vi "Status.vi"() -> ()   [LabVIEW 2013]
uses:
  Arm Globals.vi
  ROS/Code/Console/Servers/ServerSubs/(nist) Arm Globals.vi
panel:
  out "L: End":bool caption="Abort"
  out "L: Pause":bool caption="Pause"
  out "L: Status":string="Initial" caption="Prim Status"
  in  "Use Through Point":bool=TRUE
  in  "Zero V":bool
  out "R: End":bool caption="Abort"
  out "R: Pause":bool caption="Pause"
  in  "stop":bool
  out "R:Status":string="Home" caption="Prim Status"
  # "Right"
  # "Left"
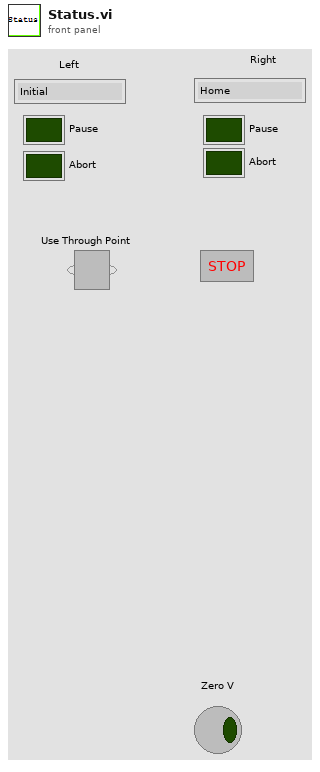
[diagram p1: front panel]
types:
  T1 = cluster{"Label":string, "Arm Angles (degrees)":dbl[]}
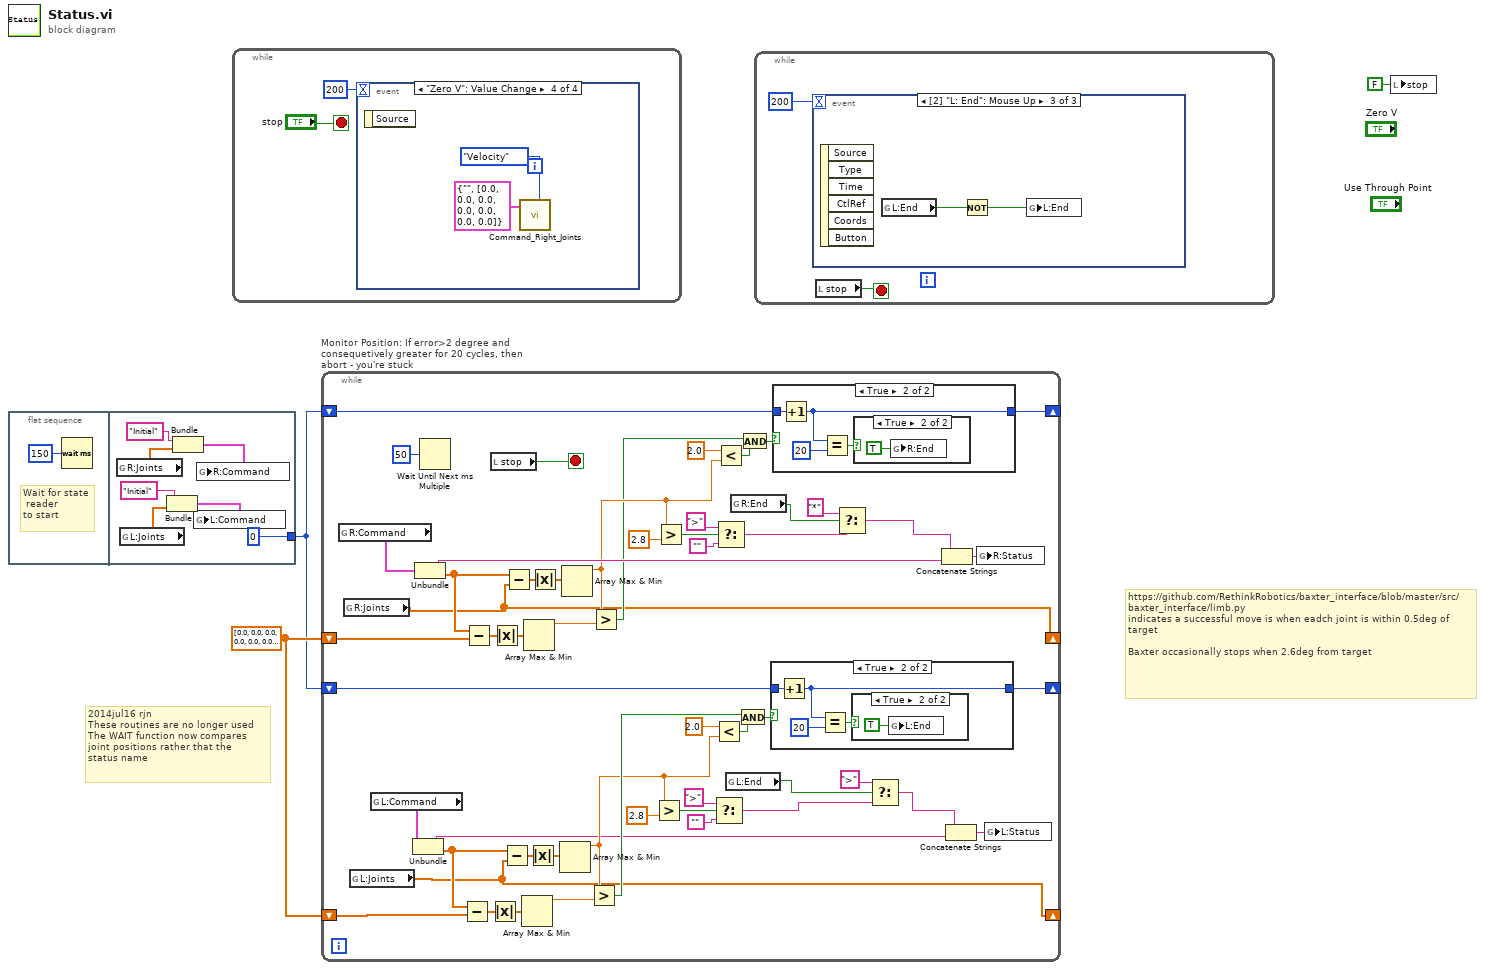
[diagram p0: block diagram]
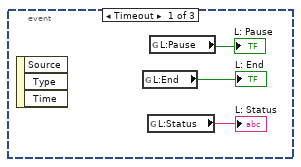
[diagram p2: hidden frame]
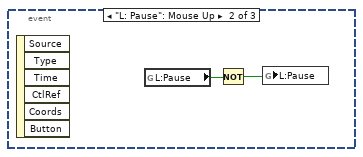
[diagram p3: hidden frame]
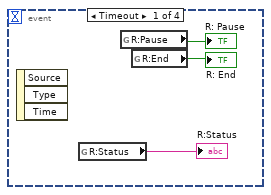
[diagram p4: hidden frame]
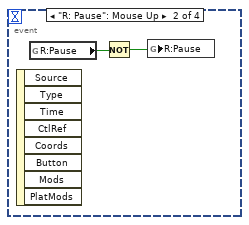
[diagram p5: hidden frame]
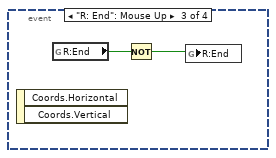
[diagram p6: hidden frame]
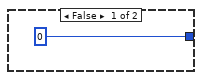
[diagram p7: hidden frame]
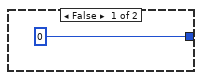
[diagram p9: hidden frame]
diagram:
  w2 = dbl[] [0.0, 0.0, 0.0, 0.0, 0.0, 0.0, 0.0] ("Positions")
  # "2014jul16 rjn\nThese routines are no longer used\nThe WAIT function now compares\njoint positions rather that the \nstatus name"
  # "https://github.com/RethinkRobotics/baxter_interface/blob/master/src/baxter_interface/limb.py\nindicates a successful move is when eadch joint is within 0.5deg of target\n\nBaxter occasionally stops when 2.6deg from target"
  n1 = flat-sequence {
    tunnel: [0] -> w1
    frame #0 {
      # "Wait for state\n reader\nto start"
      n2 = Wait (ms)(milliseconds to wait=u32 150) -> ()  [unwired: 1 out]
    }
    frame #1 {
      n3 = global read "(nist) Arm Globals.vi" "R:Joints"() -> (w6:dbl[])
      n4 = global read "(nist) Arm Globals.vi" "L:Joints"() -> (w5:dbl[])
      n5 = Bundle("Initial", "L:Joints"=w5) -> (w7:cluster{string, "L:Joints":dbl[]})  [unwired: 1 in]
      n6 = Bundle("Initial", "R:Joints"=w6) -> (w8:cluster{string, "R:Joints":dbl[]})  [unwired: 1 in]
      n7 = global write "Arm Globals.vi" "L:Command"(w7) -> ()
      n8 = global write "Arm Globals.vi" "R:Command"(w8) -> ()
    }
  }
  n9 = while {
    stop <- "stop" stop-if-true
    n10 = event shown="[3] \"Zero V\": Value Change" {
      selector: _ -> [_ _ _ _]
      dyn-events: _ -> [_ _ _ _]
      timeout: 200 -> [_ _ _ _]
      event Timeout {
        n11 = event-data() -> ()  [unwired: 1 in, 3 out]
        n12 = global read "Arm Globals.vi" "R:Status"() -> (→"R:Status":string)
        n13 = global read "Arm Globals.vi" "R:Pause"() -> (→"R: Pause":bool)
        n14 = global read "Arm Globals.vi" "R:End"() -> (→"R: End":bool)
      }
      event "R: Pause": Mouse Up {
        n15 = event-data() -> ()  [unwired: 1 in, 8 out]
        n16 = global read "Arm Globals.vi" "R:Pause"() -> (w18:bool)
        n17 = Not(x=w18) -> (.not. x?=w17:bool)
        n18 = global write "Arm Globals.vi" "R:Pause"(w17) -> ()
      }
      event "R: End": Mouse Up {
        n19 = event-data() -> ()  [unwired: 1 in, 2 out]
        n20 = global read "Arm Globals.vi" "R:End"() -> (w20:bool)
        n21 = Not(x=w20) -> (.not. x?=w19:bool)
        n22 = global write "Arm Globals.vi" "R:End"(w19) -> ()
      }
      event "Zero V": Value Change {
        n23 = event-data() -> ()  [unwired: 1 in, 1 out]
        n24 = call "Command_Right_Joints.vi"("Mode"=enum32{"Position", "Velocity", "Effort"}."Velocity", "Goal"=T1 {"Label"="", "Arm Angles (degrees)"=[0.0, 0.0, 0.0, 0.0, 0.0, 0.0, 0.0]}) -> ()  [unwired: 6 in, 2 out]
      }
    }
  }
  n25 = while "Monitor Position: If error>2 degree and consequetively greater for 20 cycles, then abort - you're stuck" {
    shift-right: [w73] -> _
    shift-left: w1 -> [w72]
    shift-right: [w24] -> _
    shift-left: w2 -> [w59]
    shift-right: [w35] -> _
    shift-left: w1 -> [w36]
    shift-right: [w23] -> _
    shift-left: w2 -> [w37]
    stop <- w71 stop-if-true
    n26 = global read "Arm Globals.vi" "R:Command"() -> (w26:cluster{"Label":string, "Angles":dbl[]})
    n27 = global read "(nist) Arm Globals.vi" "R:Joints"() -> (w24:dbl[])
    n28 = global read "(nist) Arm Globals.vi" "L:Joints"() -> (w23:dbl[])
    n29 = global read "Arm Globals.vi" "L:Command"() -> (w25:cluster{"Label":string, "Angles":dbl[]})
    n30 = Unbundle(w25) -> ("Label"=w45:string, "Angles"=w50:dbl[])
    n31 = Unbundle(w26) -> ("Label"=w65:string, "Angles"=w60:dbl[])
    n32 = Wait Until Next ms Multiple(millisecond multiple=u32 50) -> ()  [unwired: 1 out]
    n33 = Subtract(x=w50, y=w37) -> (x-y=w51:dbl[])
    n34 = Subtract(x=w60, y=w59) -> (x-y=w58:dbl[])
    n35 = Absolute Value(x=w51) -> (abs(x)=w49:dbl[])
    n36 = local read "stop"() -> (w71:bool)
    n37 = Absolute Value(x=w58) -> (abs(x)=w61:dbl[])
    n38 = Subtract(x=w50, y=w23) -> (x-y=w38:dbl[])
    n39 = Subtract(x=w60, y=w24) -> (x-y=w76:dbl[])
    n40 = Array Max & Min(array=w49) -> (max value=w52:dbl)  [unwired: 3 out]
    n41 = Array Max & Min(array=w61) -> (max value=w57:dbl)  [unwired: 3 out]
    n42 = Absolute Value(x=w38) -> (abs(x)=w40:dbl[])
    n43 = Absolute Value(x=w76) -> (abs(x)=w70:dbl[])
    n44 = Array Max & Min(array=w40) -> (max value=w53:dbl)  [unwired: 3 out]
    n45 = Array Max & Min(array=w70) -> (max value=w56:dbl)  [unwired: 3 out]
    n46 = Greater?(x=w53, y=w52) -> (0:w54:bool)
    n47 = Greater?(x=w56, y=w57) -> (0:w55:bool)
    n48 = Greater?(x=w53, y=2.8) -> (0:w42:bool)
    n49 = Greater?(x=w56, y=2.8) -> (0:w68:bool)
    n50 = Less?(x=2.0, y=w53) -> (x < y?=w47:bool)
    n51 = Select(t=">", s=w42, f="") -> (s? t:f=w30:string)
    n52 = Less?(x=2.0, y=w56) -> (x < y?=w63:bool)
    n53 = Select(t=">", s=w68, f="") -> (s? t:f=w33:string)
    n54 = global read "Arm Globals.vi" "L:End"() -> (w29:bool)
    n55 = global read "Arm Globals.vi" "R:End"() -> (w32:bool)
    n56 = And(x=w54, y=w47) -> (x .and. y?=w48:bool)
    n57 = And(x=w55, y=w63) -> (x .and. y?=w62:bool)
    n58 = case shown="True" w48 {
      tunnel: [0 w80] -> w35
      tunnel: w36 -> [_ w81]
      frame False {
      }
      frame True {
        n59 = Increment(x=w81) -> (x+1=w80:i32)
        n60 = Equal?(x=w80, y=20) -> (x = y?=w78:bool)
        n61 = case shown="True" w78 {
          frame False {
          }
          frame True {
            n62 = global write "Arm Globals.vi" "L:End"(TRUE ("L:End")) -> ()
          }
        }
      }
    }
    n63 = case shown="True" w62 {
      tunnel: [0 w86] -> w73
      tunnel: w72 -> [_ w87]
      frame False {
      }
      frame True {
        n64 = Increment(x=w87) -> (x+1=w86:i32)
        n65 = Equal?(x=w86, y=20) -> (x = y?=w84:bool)
        n66 = case shown="True" w84 {
          frame False {
          }
          frame True {
            n67 = global write "Arm Globals.vi" "R:End"(TRUE ("R:End")) -> ()
          }
        }
      }
    }
    n68 = Select(t="*", s=w32, f=w33) -> (s? t:f=w31:string)
    n69 = Select(t=">", s=w29, f=w30) -> (s? t:f=w27:string)
    n70 = Concatenate Strings(w31, w65) -> (w64:string)
    n71 = Concatenate Strings(w27, w45) -> (w46:string)
    n72 = global write "Arm Globals.vi" "R:Status"(w64) -> ()
    n73 = global write "Arm Globals.vi" "L:Status"(w46) -> ()
  }
  n74 = while {
    stop <- w90 stop-if-true
    n75 = event shown="[2] \"L: End\": Mouse Up" {
      selector: _ -> [_ _ _]
      dyn-events: _ -> [_ _ _]
      timeout: 200 -> [_ _ _]
      event Timeout {
        n76 = event-data() -> ()  [unwired: 1 in, 3 out]
        n77 = global read "Arm Globals.vi" "L:End"() -> (→"L: End":bool)
        n78 = global read "Arm Globals.vi" "L:Status"() -> (→"L: Status":string)
        n79 = global read "Arm Globals.vi" "L:Pause"() -> (→"L: Pause":bool)
      }
      event "L: Pause": Mouse Up {
        n80 = event-data() -> ()  [unwired: 1 in, 6 out]
        n81 = global read "Arm Globals.vi" "L:Pause"() -> (w94:bool)
        n82 = Not(x=w94) -> (.not. x?=w95:bool)
        n83 = global write "Arm Globals.vi" "L:Pause"(w95) -> ()
      }
      event "L: End": Mouse Up {
        n84 = event-data() -> ()  [unwired: 1 in, 6 out]
        n85 = global read "Arm Globals.vi" "L:End"() -> (w97:bool)
        n86 = Not(x=w97) -> (.not. x?=w96:bool)
        n87 = global write "Arm Globals.vi" "L:End"(w96) -> ()
      }
    }
    n88 = local read "stop"() -> (w90:bool)
  }
  n89 = local write "stop"(FALSE ("stop")) -> ()
